vi "CV Voltage Limits.vi"(11 "CV Voltage In":dbl[](array[numeric])) -> (3 "CV Voltage Out":dbl[](array[numeric]))   [LabVIEW 2018]
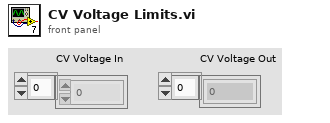
[diagram p1: front panel]
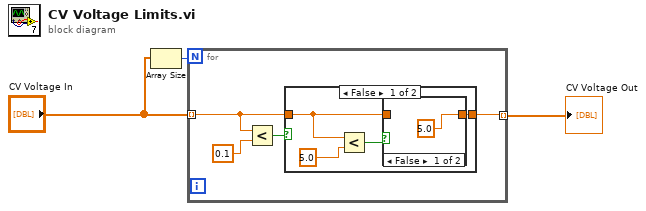
[diagram p0: block diagram]
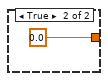
[diagram p3: hidden frame]
diagram:
  n1 = Array Size(array="CV Voltage In") -> (size(s)=w1:i32)
  n2 = for {
    N: w1 -> [_]
    tunnel: "CV Voltage In" -> [w4] mode=indexing
    tunnel: [w5] -> w3 mode=indexing
    n3 = Less?(x=w4, y=0.1) -> (x < y?=w7:bool)
    n4 = case shown="False" w7 {
      tunnel: w4 -> [w9 _]
      tunnel: [w8 0.0 ("y")] -> w5
      frame False {
        n5 = Less?(x=w9, y=5.0) -> (x < y?=w11:bool)
        n6 = case shown="False" w11 {
          tunnel: w9 -> [_ w13]
          tunnel: [5.0 ("y") w13] -> w8
          frame False {
          }
          frame True {
          }
        }
      }
      frame True {
      }
    }
  }
  "CV Voltage Out" <- w3
